vi "UI.Connection.State.Get.vi"(6 "Menu Ref":refnum<k9>, 8 "error in (no error)":errorcluster, 11 "State Variables":T1) -> (0 "error out":errorcluster, 1 "Addon Connected?":bool, 3 "State Variables out":T1)   [LabVIEW 2019, in "Ghost Bus Workspace Shared.lvlib"]
uses:
  Ghost Bus Workspace Shared.lvlib
  <vilib>/NI VeriStand/Execution/Workspace/WorkspaceAPI.ctl
  NationalInstruments.VeriStand.ClientAPI
  NationalInstruments.VeriStand.SystemDefinitionAPI
  <vilib>/NI VeriStand/Execution/Workspace/NI_VS Workspace ExecutionAPI.lvlib
  NationalInstruments.VeriStand.SystemStorage
  Types/Workspace.SavedState.ctl
  <vilib>/NI VeriStand/Display Template Support/DisplayTemplateSupport.llb/enum_Display Template Handler Minimal To Workspace.ctl
  <vilib>/NI VeriStand/Execution/Workspace/Target State.ctl
  <vilib>/NI VeriStand/Execution/Workspace/Target State Info.ctl
  <vilib>/NI VeriStand/Execution/Workspace/SystemStateRegEventRef.ctl
  <vilib>/NI VeriStand/Display Template Support/DisplayTemplateSupport.llb/enum_Display Template Handler Minimal To Widget Msg.ctl
  <vilib>/NI VeriStand/Execution/Workspace/SystemStateEventRef.ctl
  SubModules/CAN-Streaming-Support/Source/Addon/Addon Shared/Types/Type Filter.ctl
  SubModules/CAN-Streaming-Support/Source/Addon/Addon Shared/CAN Stream Support Shared.lvlib
  Types/UI.Refs.ctl
  SubModules/CAN-Streaming-Support/Source/UIs/Workspace Shared/Types/Host Stream Queue Command.ctl
  SubModules/CAN-Streaming-Support/Source/UIs/Workspace Shared/CAN Stream Support Workspace Shared.lvlib
  SubModules/CAN-Streaming-Support/Source/UIs/Workspace Shared/Types/Host Stream Queue Type.ctl
  <vilib>/xnet/xnet.llb/XNET Frame Type CAN.ctl
  <vilib>/xnet/xnet.llb/XNET Frame CAN.ctl
  SubModules/CAN-Streaming-Support/Source/UIs/Workspace Shared/Types/Host Stream Queue Refs.ctl
  Types/Workspace.State.ctl
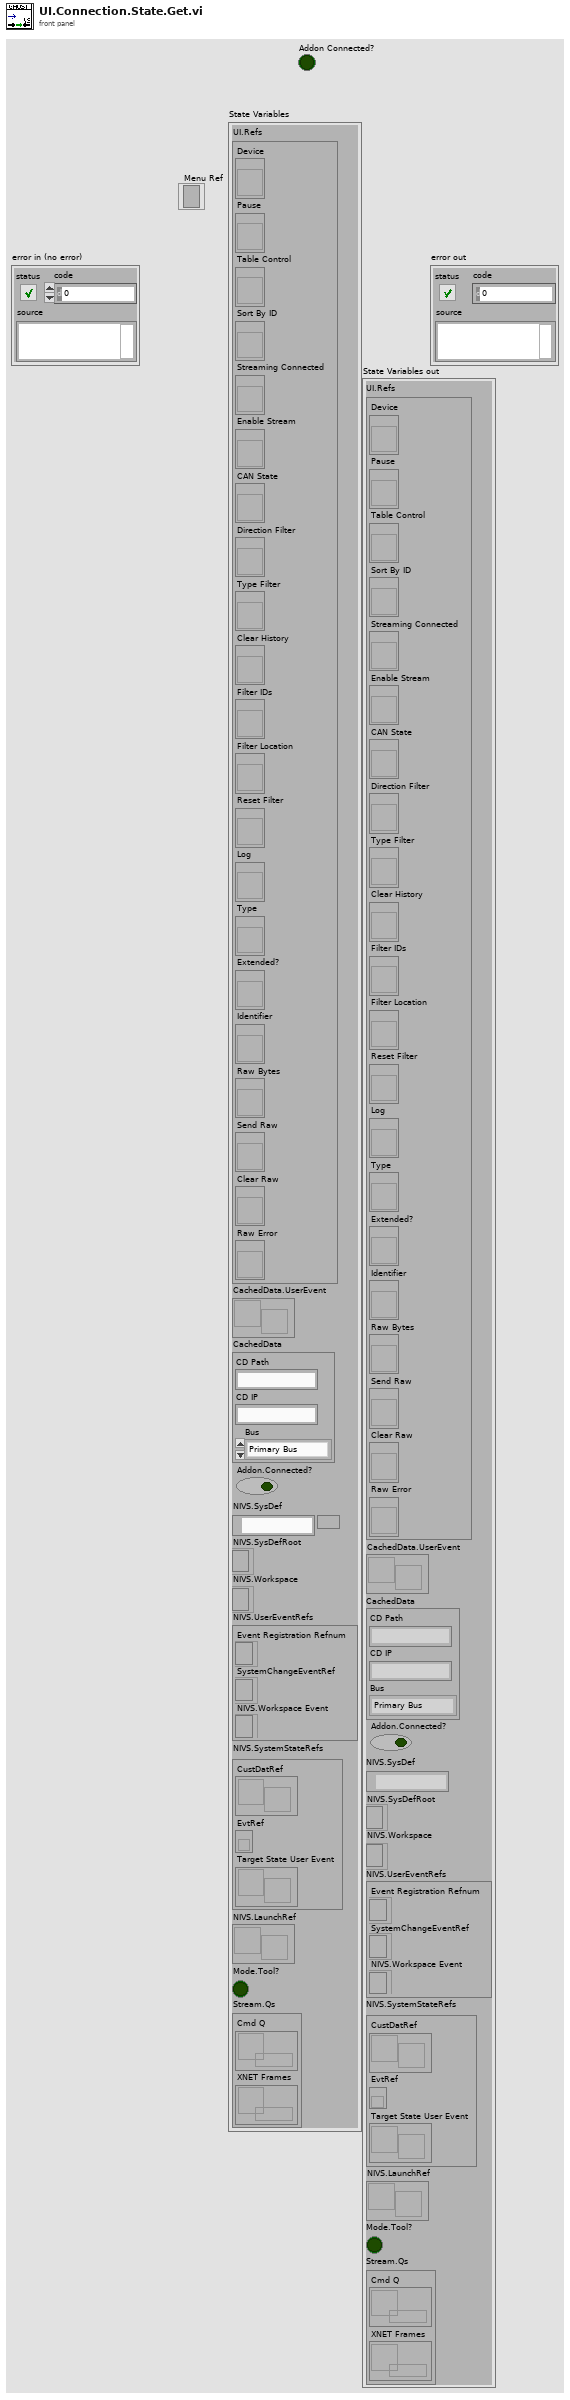
[diagram p1: front panel]
types:
  T1 = typedef "Ghost Bus Workspace Shared.lvlib/Workspace.State.ctl" = cluster{"UI.Refs":T2, "CachedData.UserEvent":refnum<user-event>, "CachedData":T3, "Addon.Connected?":bool, "NIVS.SysDef":path, "NIVS.SysDefRoot":refnum<k24>, "NIVS.Workspace":T4, "NIVS.UserEventRefs":cluster{"Event Registration Refnum":refnum<event-registration>, "SystemChangeEventRef":T5, "NIVS.Workspace Event":refnum<event-registration>}, "NIVS.SystemStateRefs":T6, "NIVS.LaunchRef":refnum<user-event>, "Mode.Tool?":bool, "Stream.Qs":T7}
  T2 = typedef "Ghost Bus Workspace Shared.lvlib/UI.Refs.ctl" = cluster{"Device":refnum<vi>, "Pause":refnum<vi>, "Table Control":refnum<vi>, "Sort By ID":refnum<vi>, "Streaming Connected":refnum<vi>, "Enable Stream":refnum<vi>, "CAN State":refnum<vi>, "Direction Filter":refnum<vi>, "Type Filter":refnum<vi>, "Clear History":refnum<vi>, "Filter IDs":refnum<vi>, "Filter Location":refnum<vi>, "Reset Filter":refnum<vi>, "Log":refnum<vi>, "Type":refnum<vi>, "Extended?":refnum<vi>, "Identifier":refnum<vi>, "Raw Bytes":refnum<vi>, "Send Raw":refnum<vi>, "Clear Raw":refnum<vi>, "Raw Error":refnum<vi>}
  T3 = typedef "Ghost Bus Workspace Shared.lvlib/Workspace.SavedState.ctl" = cluster{"CD Path":string, "CD IP":string, "Bus":enum16{"Primary Bus", "Ghost Bus"}}
  T4 = typedef "NI_VS Workspace ExecutionAPI.lvlib/WorkspaceAPI.ctl" = refnum<k24>
  T5 = typedef "NI_VS Workspace ExecutionAPI.lvlib/SystemStateRegEventRef.ctl" = refnum<event-registration>
  T6 = typedef "NI_VS Workspace ExecutionAPI.lvlib/SystemStateEventRef.ctl" = cluster{"CustDatRef":refnum<user-event>, "EvtRef":refnum<k27>, "Target State User Event":refnum<user-event>}
  T7 = typedef "CAN Stream Support Workspace Shared.lvlib/Host Stream Queue Refs.ctl" = cluster{"Cmd Q":refnum<queue>, "XNET Frames":refnum<queue>}
  T8 = typedef "NI_VS Workspace ExecutionAPI.lvlib/SystemState.ctl" = u8
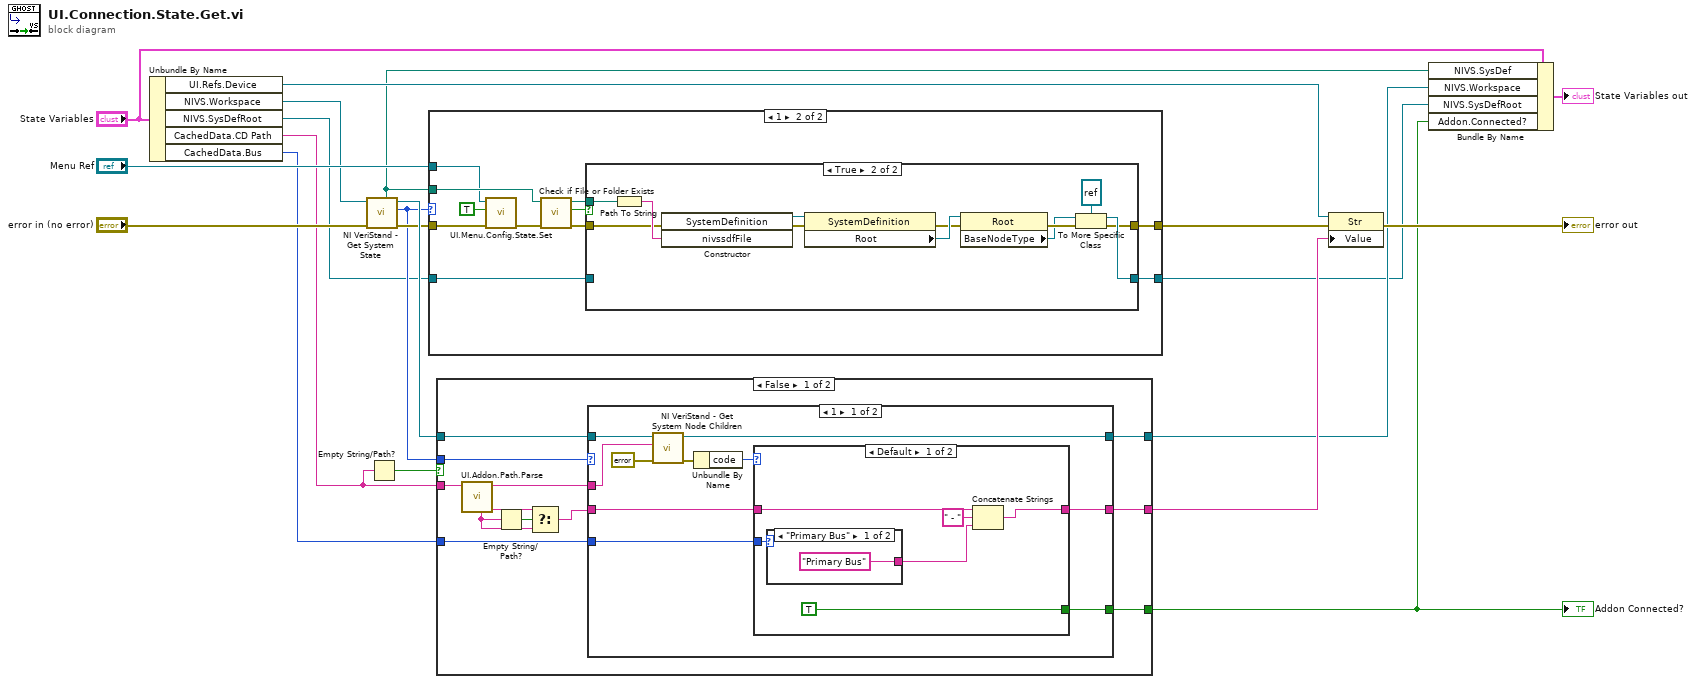
[diagram p0: block diagram]
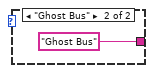
[diagram p2: hidden frame]
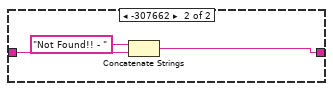
[diagram p3: hidden frame]
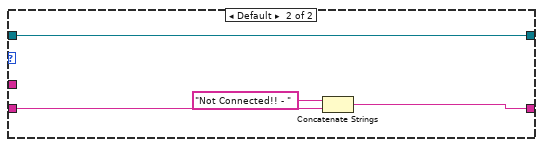
[diagram p4: hidden frame]
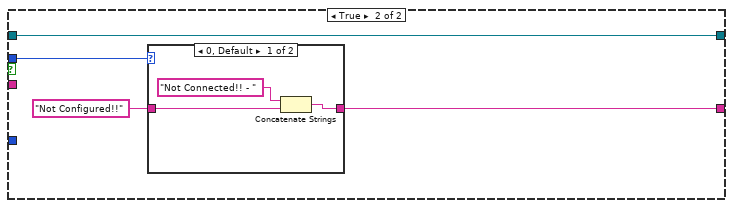
[diagram p5: hidden frame]
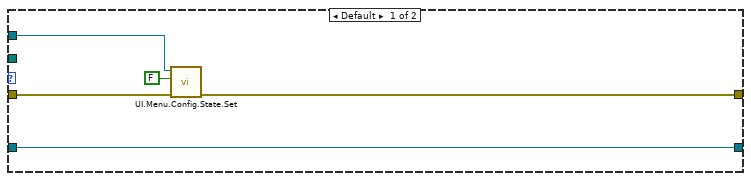
[diagram p7: hidden frame]
diagram:
  n1 = Unbundle By Name("State Variables") -> ("UI.Refs.Device"=w11:refnum<vi>, "NIVS.Workspace"=w10:T4, "NIVS.SysDefRoot"=w9:refnum<k24>, "CachedData.CD Path"=w8:string, "CachedData.Bus"=w1:enum16{"Primary Bus", "Ghost Bus"})
  n2 = call <vilib>:"NI VeriStand - Get System State.vi"("error in (no error)"="error in (no error)", "WorkspaceManager in"=w10) -> ("error out"=w15:errorcluster, "System State"=w13:T8, "WorkspaceManager  out"=w16:T4, "System Definition File"=w4:path)  [unwired: 5 in, 1 out]
  n3 = Empty String/Path?(string/path=w8) -> (empty?=w20:bool)
  n4 = case shown="1" w13 {
    tunnel: [w25 w36] -> w3
    tunnel: [w23 w35] -> w14
    tunnel: w9 -> [w25 w32]
    tunnel: w15 -> [w22 w27]
    tunnel: w4 -> [_ w31]
    tunnel: "Menu Ref" -> [w21 w26]
    frame Default {
      n5 = call "UI.Menu.Config.State.Set.vi"("error in (no error)"=w22, "Enabled"=FALSE, "menu reference"=w21) -> ("error out"=w23:errorcluster)  [unwired: 8 in]
    }
    frame 1 {
      n6 = call "UI.Menu.Config.State.Set.vi"("error in (no error)"=w27, "Enabled"=TRUE, "menu reference"=w26) -> ("error out"=w28:errorcluster)  [unwired: 8 in]
      n7 = call <vilib>:"Check if File or Folder Exists.vi"("error in (no error)"=w28, "path"=w31) -> ("error out"=w34:errorcluster, "file or folder exists?"=w33:bool, "dup path"=w30:path)  [unwired: 7 in]
      n8 = case shown="True" w33 {
        tunnel: [w37 w40] -> w36
        tunnel: [w38 w39] -> w35
        tunnel: w34 -> [w38 w47]
        tunnel: w30 -> [_ w46]
        tunnel: w32 -> [w37 _]
        frame False {
        }
        frame True {
          n9 = Path To String(path=w46) -> (string=w49:string)
          n10 = constructor class="SystemDefinition"(error in=w47, "nivssdfFile"=w49) -> (reference out=w50:refnum<k24>, error out=w48:errorcluster)  [unwired: 2 in, 2 out]
          n11 = property class="SystemDefinition"(reference=w50, error in=w48) -> (error out=w41:errorcluster, "Root"=w42:refnum<k24>)  [unwired: 1 out]
          n12 = property class="Root"(reference=w42, error in=w41) -> (error out=w45:errorcluster, "BaseNodeType"=w44:refnum<k24>)  [unwired: 1 out]
          n13 = To More Specific Class(target class=refnum<k24> refnum, reference=w44, error in=w45) -> (specific class reference=w40:refnum<k24>, error out=w39:errorcluster)
        }
      }
    }
  }
  n14 = case shown="False" w20 {
    tunnel: [w62 w88] -> w19
    tunnel: [w61 w91] -> w5
    tunnel: w8 -> [w57 _]
    tunnel: [w60 _] -> w6
    tunnel: w13 -> [w58 w90]
    tunnel: w16 -> [w59 w91]
    tunnel: w1 -> [w51 _]
    frame False {
      n15 = call "UI.Addon.Path.Parse.vi"("Cached Addon Path"=w57) -> ("Addon Name"=w53:string, "Addon Path"=w56:string, "Remaining Path"=w54:string)  [unwired: 6 in, 2 out]
      n16 = Empty String/Path?(string/path=w54) -> (empty?=w55:bool)
      n17 = Select(t=w53, s=w55, f=w54) -> (s? t:f=w52:string)
      n18 = case shown="1" w58 {
        tunnel: [w72 w87] -> w62
        tunnel: w52 -> [w71 w85]
        tunnel: [w68 w86] -> w61
        tunnel: [w67 _] -> w60
        tunnel: w59 -> [w66 w86]
        tunnel: w56 -> [w64 _]
        tunnel: w51 -> [w63 _]
        frame 1 {
          n19 = call <vilib>:"NI VeriStand - Get System Node Children.vi"("error in (no error)"=errorcluster {"status"=FALSE, "code"=0, "source"=""}, "Node"=w64, "WorkspaceManager in"=w66) -> ("error out"=w70:errorcluster, "WorkspaceManager out"=w68:T4)  [unwired: 6 in, 1 out]
          n20 = Unbundle By Name(w70) -> ("code"=w69:i32)
          n21 = case shown="Default" w69 {
            tunnel: w71 -> [w74 w82]
            tunnel: [w75 w83] -> w72
            tunnel: [TRUE _] -> w67
            tunnel: w63 -> [w77 _]
            frame Default {
              n22 = case shown="\"Primary Bus\"" w77 {
                tunnel: ["Primary Bus" ("string") "Ghost Bus" ("string")] -> w73
                frame "Primary Bus" {
                }
                frame "Ghost Bus" {
                }
              }
              n23 = Concatenate Strings(w74, " - " ("string"), w73) -> (w75:string)
            }
            frame -307662 {
              n24 = Concatenate Strings("Not Found!! - " ("string"), w82) -> (w83:string)
            }
          }
        }
        frame Default {
          n25 = Concatenate Strings("Not Connected!! - " ("string"), w85) -> (w87:string)
        }
      }
    }
    frame True {
      n26 = case shown="0, Default" w90 {
        tunnel: [w93 w95] -> w88
        tunnel: "Not Configured!!" ("CD Path in") -> [w94 w95]
        frame 0, Default {
          n27 = Concatenate Strings("Not Connected!! - " ("string"), w94) -> (w93:string)
        }
        frame 1 {
        }
      }
    }
  }
  "Addon Connected?" <- w6
  n28 = property class="Str"(reference=w11, error in=w14, "Value"=w19) -> (error out=→"error out":errorcluster)  [unwired: 1 out]
  n29 = Bundle By Name(cluster="State Variables", "NIVS.SysDef"=w4, "NIVS.Workspace"=w5, "NIVS.SysDefRoot"=w3, "Addon.Connected?"=w6) -> (→"State Variables out":T1)
